vi "readfile.vi"(10 "name or relative path":string, 11 "Relative Path":path) -> (3 "String":string)   [LabVIEW 2019]
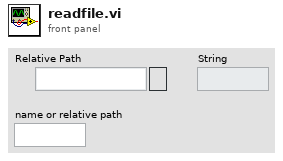
[diagram p1: front panel]
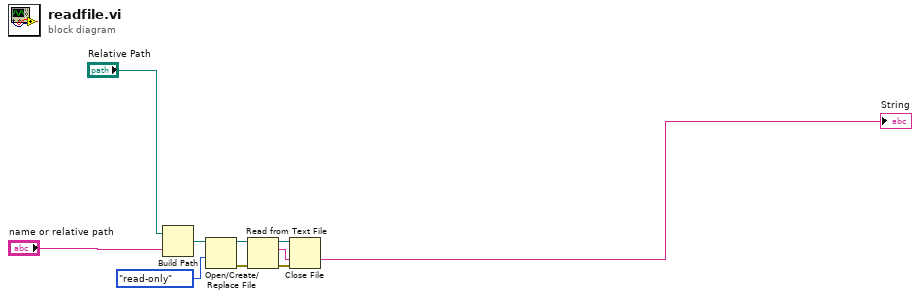
[diagram p0: block diagram]
diagram:
  n1 = Build Path(base path="Relative Path", name or relative path="name or relative path") -> (appended path=w6:path)
  n2 = Open/Create/Replace File(file path (use dialog)=w6, access (0:read/write)=enum16{"read/write", "read-only", "write-only"}."read-only") -> (refnum out=w2:refnum<file>, error out=w3:errorcluster)  [unwired: 4 in, 1 out]
  n3 = Read from Text File(file (use dialog)=w2, error in=w3) -> (refnum out=w4:refnum<file>, text=→"String":string, error out=w5:errorcluster)  [unwired: 2 in, 1 out]
  n4 = Close File(refnum=w4, error in=w5) -> ()  [unwired: 2 out]
